vi "Asensor_parccial.vi"() -> ()   [LabVIEW 2019]
panel:
  in  "Abierto/Cerrado":bool=TRUE
  in  "Sensor":bool
  out "Indicador_Piso":u16(ring)
  in  "Botonera 3":bool
  in  "Botonera 4":bool
  in  "Botonera 1":bool
  in  "Botonera 2":bool
  in  "Peticion_Abrir":bool
  in  "Peticion_Cerrar":bool
  in  "Subir/Bajar":bool
  in  "Automatico/Manual":bool
  in  "Start/Stop":bool
  in  "Piso inicial":i32=1 min=1 max=4
  out "Numeric 2":u8
  out "Numeric":i32
  out "Subiendo":bool
  out "Bajando":bool
  out "Sensor 4":bool
  out "Sensor 3":bool
  out "Sensor 2":bool
  out "Sensor 1":bool
  in  "Piso 3_Bajar":bool
  in  "Piso 3_Subir":bool
  in  "Piso 2_Bajar":bool
  in  "Piso 2_Subir":bool
  in  "Piso 1_Subir":bool
  in  "Piso 4_Bajar":bool
  out "Puerta":i32(ring)
  out "Posicion_asensor":i32(slide) scale=100.0..400.0
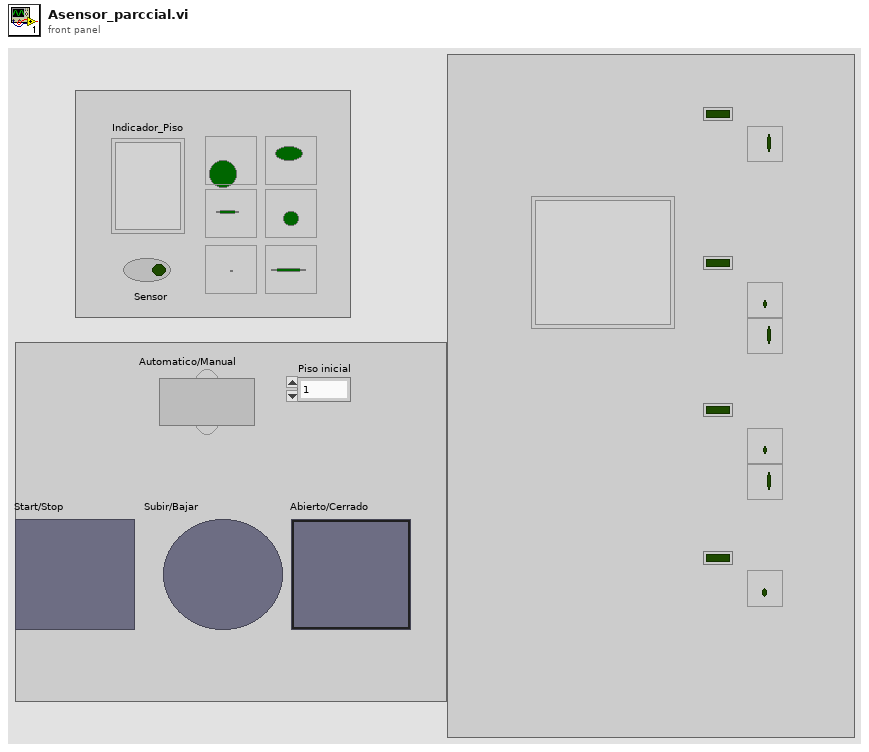
[diagram p1: front panel]
types:
  T1 = enum16{"espera", "abrir", "cerrar", "subir", "bajar"}
  T2 = enum8{"Enabled", "Disabled", "Disabled and Grayed Out"}
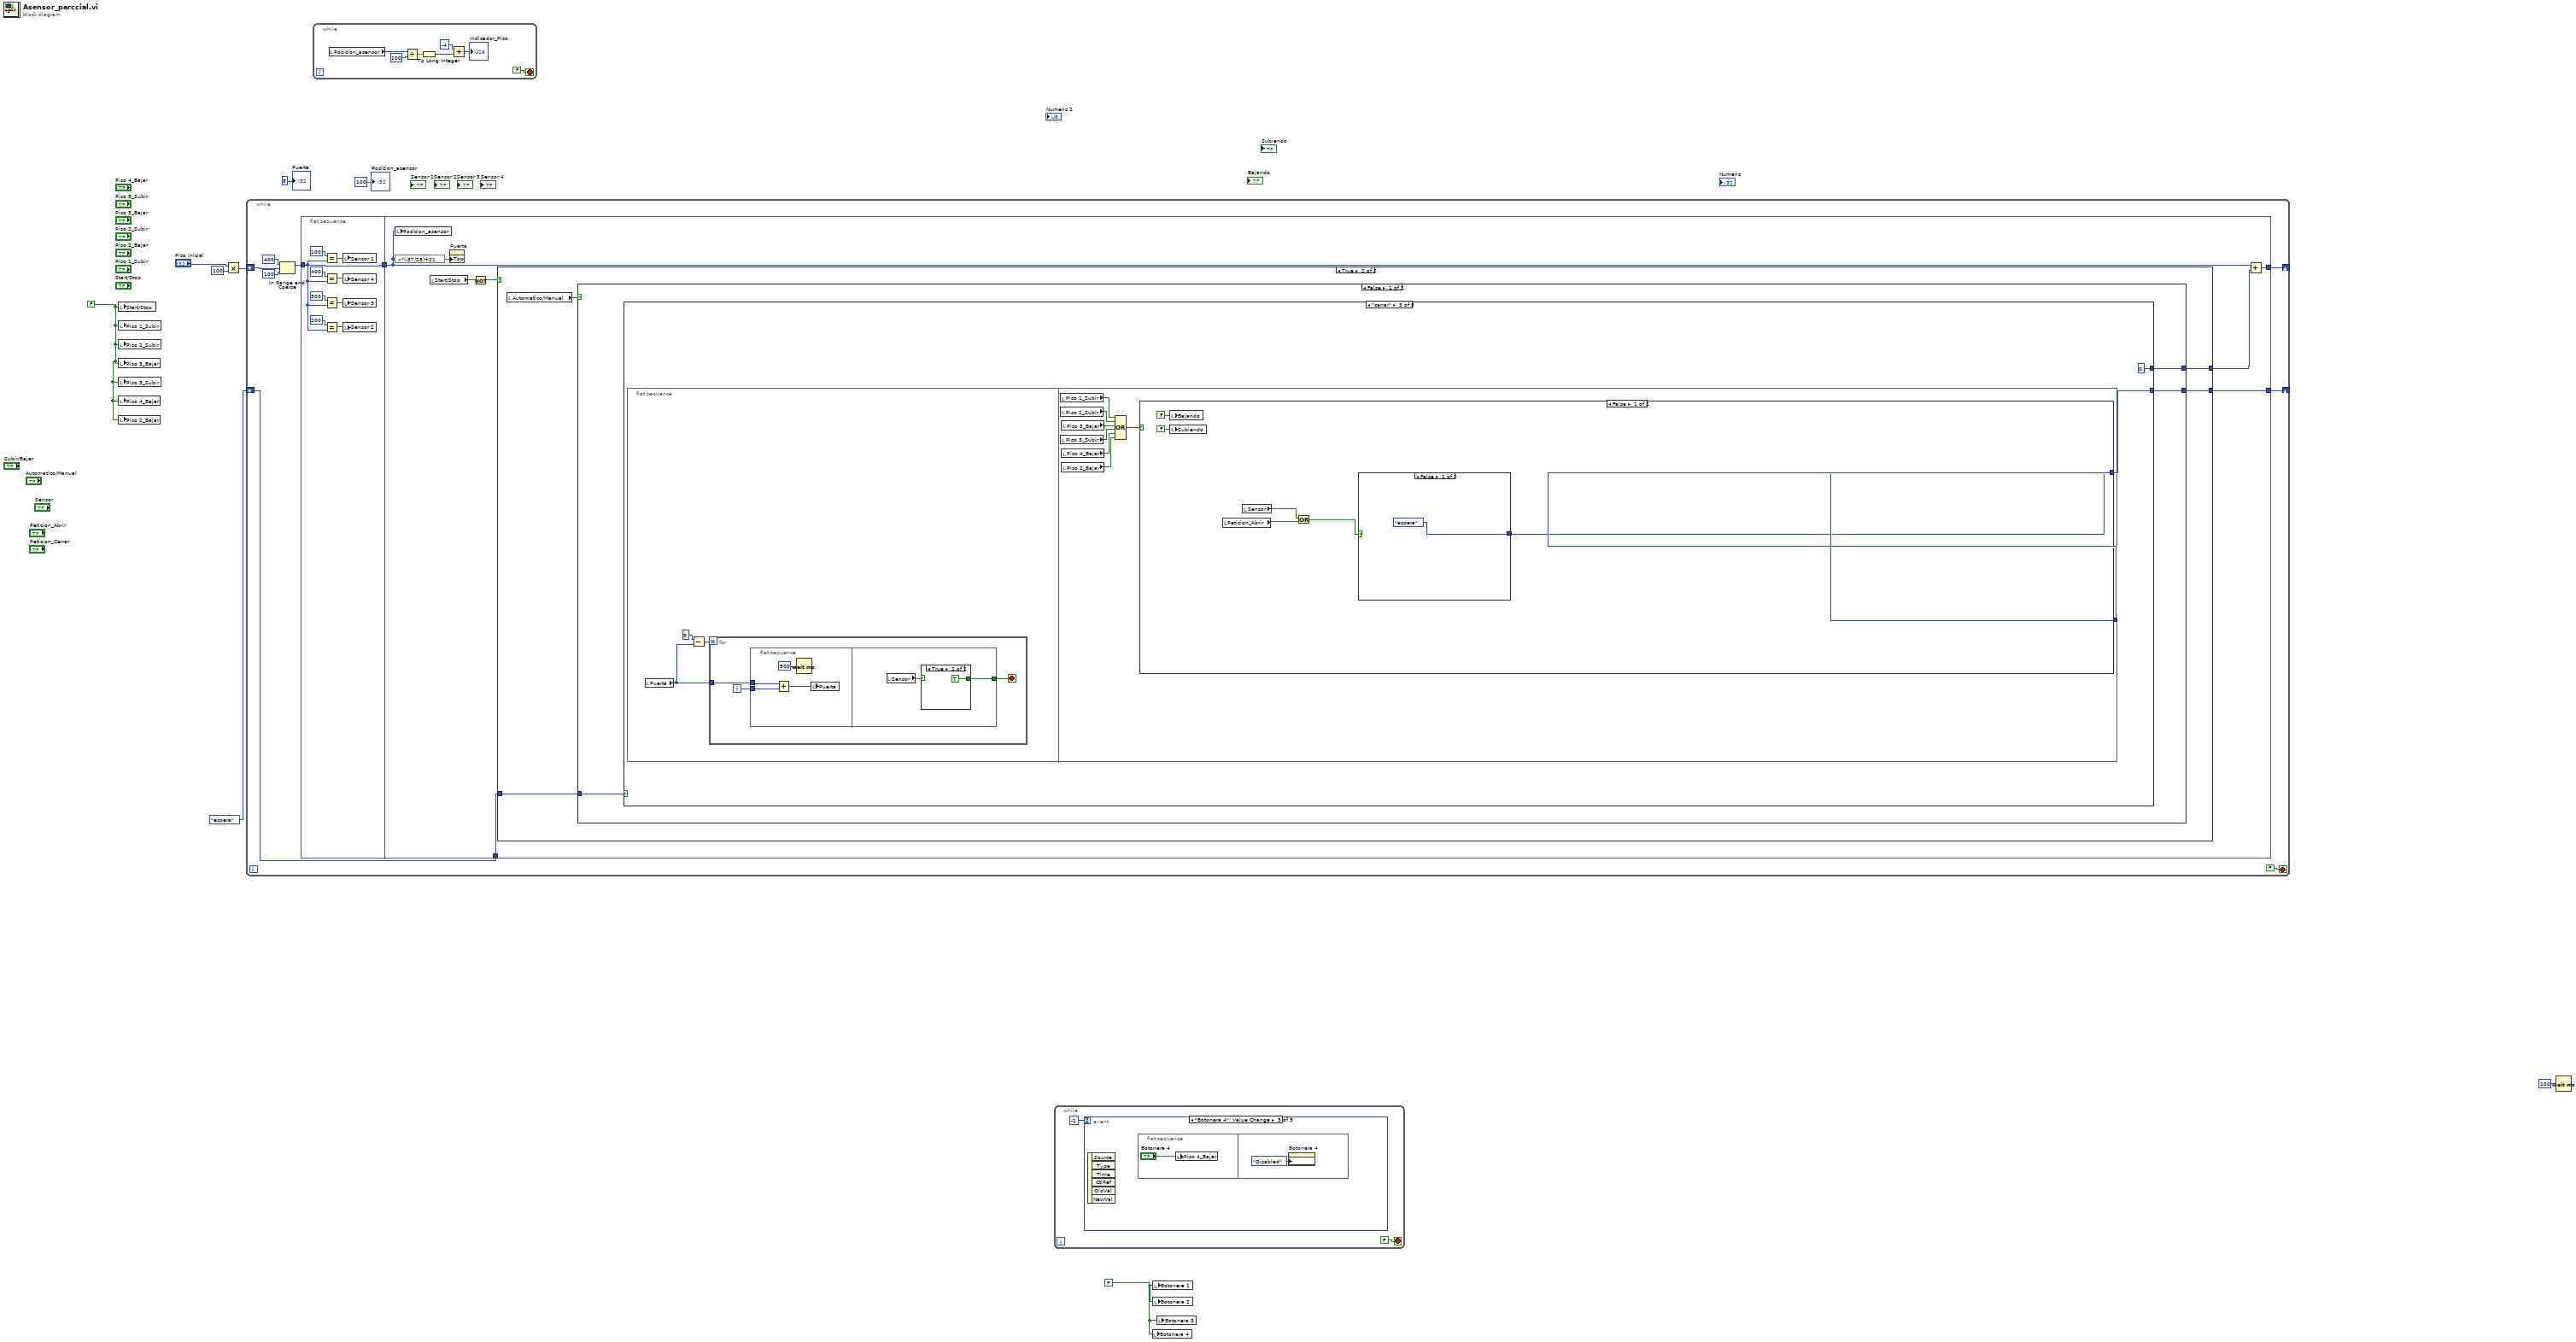
[diagram p0: block diagram]
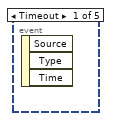
[diagram p2: hidden frame]
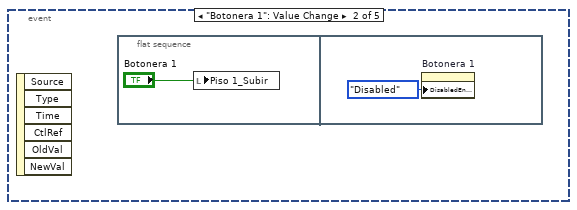
[diagram p3: hidden frame]
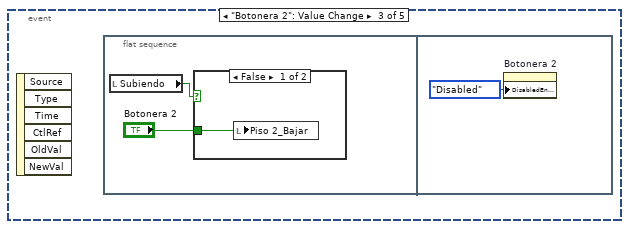
[diagram p4: hidden frame]
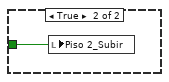
[diagram p5: hidden frame]
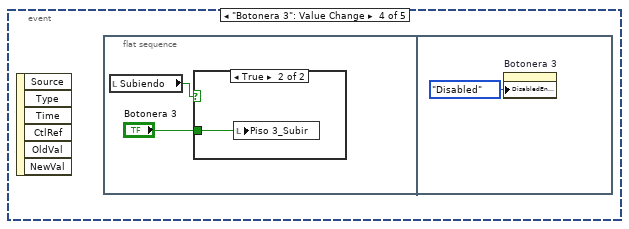
[diagram p6: hidden frame]
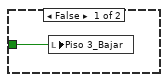
[diagram p7: hidden frame]
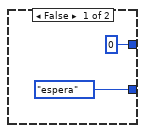
[diagram p8: hidden frame]
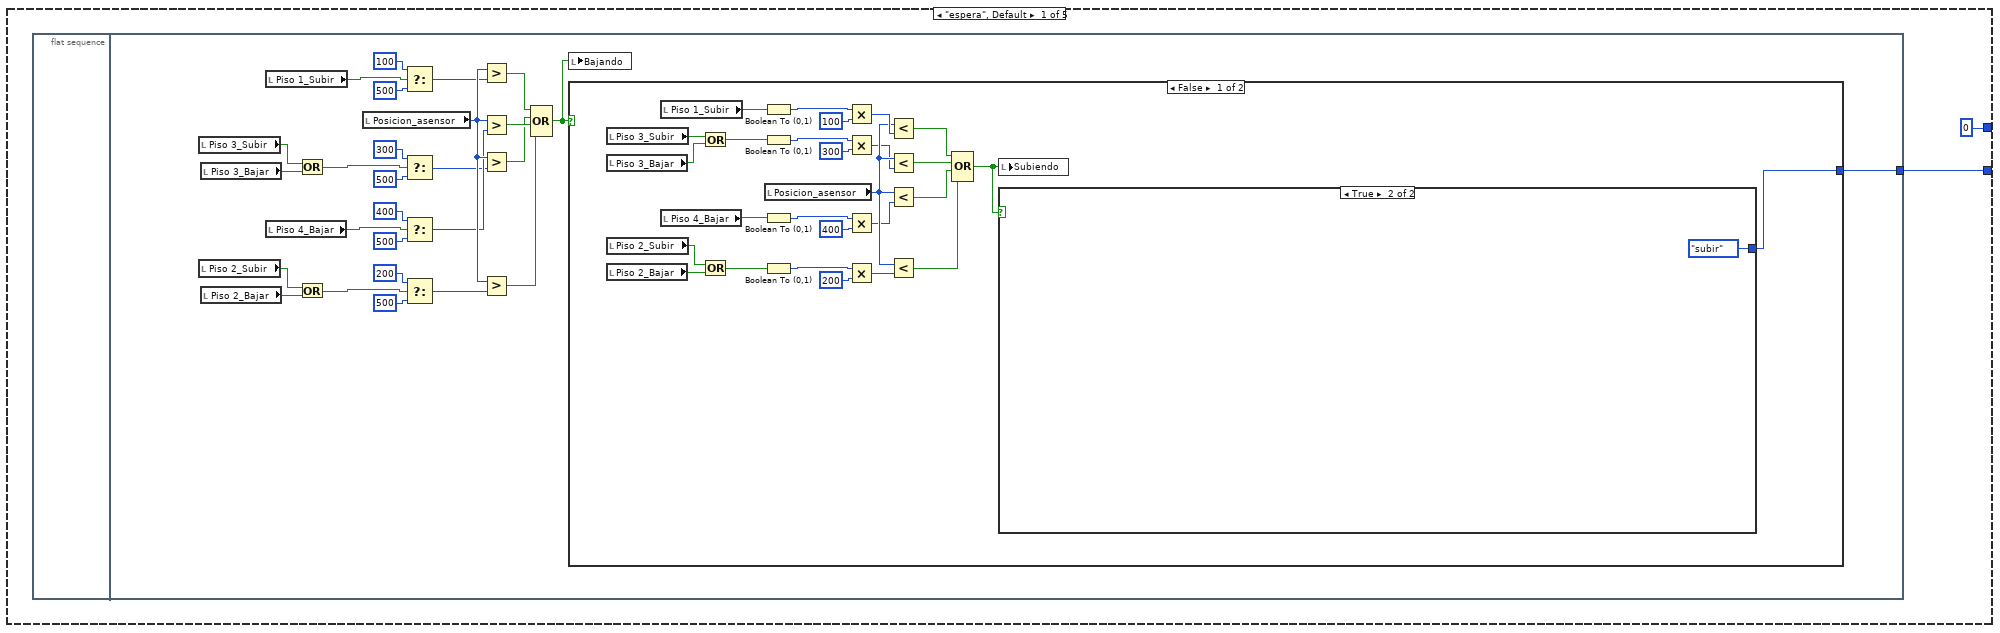
[diagram p9: hidden frame]
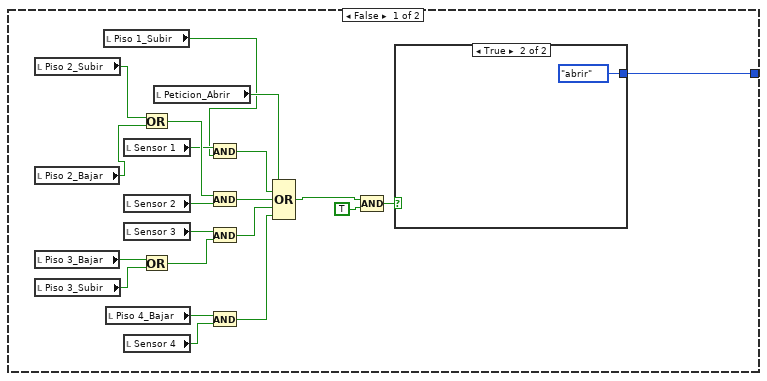
[diagram p10: hidden frame]
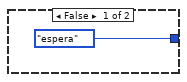
[diagram p11: hidden frame]
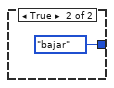
[diagram p12: hidden frame]
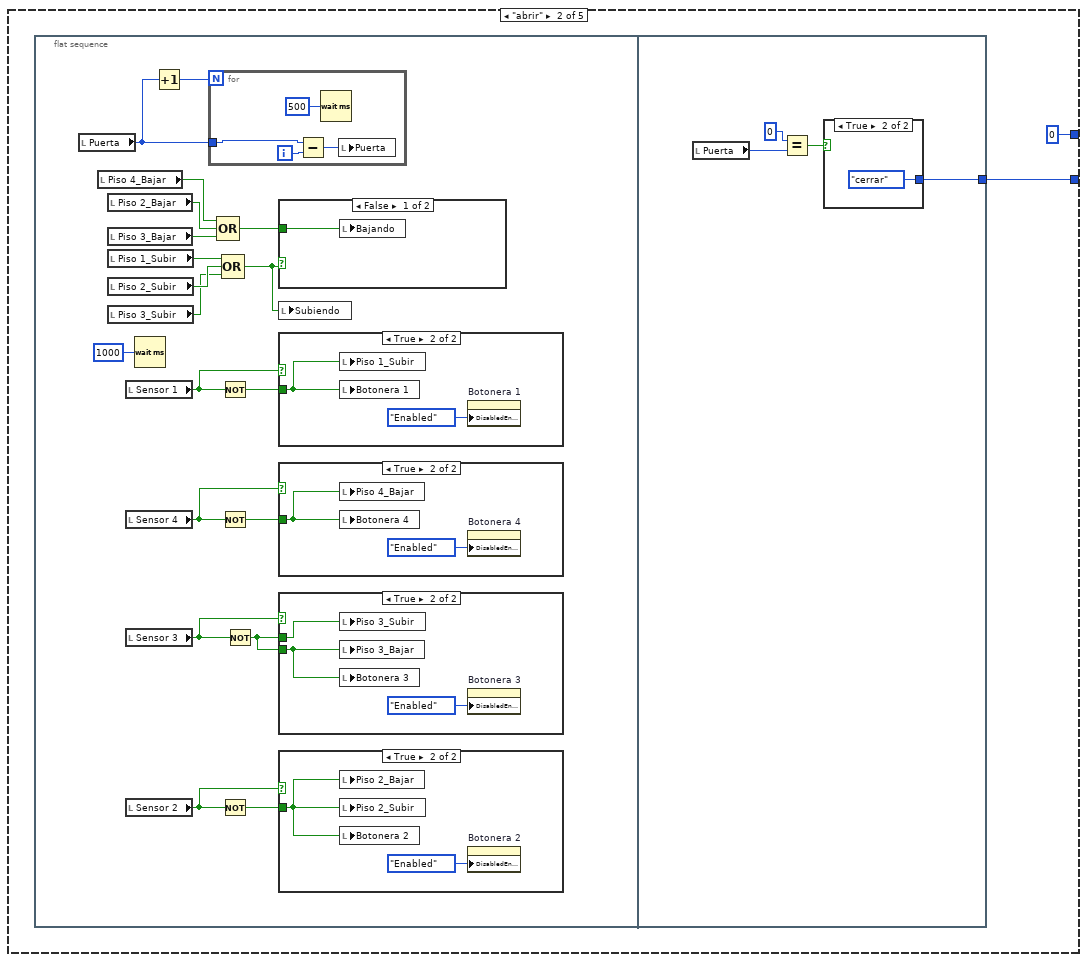
[diagram p13: hidden frame]
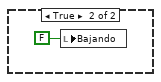
[diagram p18: hidden frame]
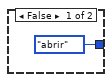
[diagram p19: hidden frame]
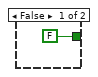
[diagram p20: hidden frame]
diagram:
  w3 = FALSE ("Botonera 1")
  w4 = FALSE ("Start/Stop")
  n1 = local write "Start/Stop"(w4) -> ()
  n2 = local write "Piso 1_Subir"(w4) -> ()
  n3 = local write "Piso 2_Subir"(w4) -> ()
  n4 = local write "Piso 3_Bajar"(w4) -> ()
  n5 = local write "Piso 3_Subir"(w4) -> ()
  n6 = local write "Piso 4_Bajar"(w4) -> ()
  n7 = local write "Piso 2_Bajar"(w4) -> ()
  n8 = Multiply(x="Piso inicial", y=100) -> (x*y=w7:i32)
  n9 = while {
    shift-right: [w12] -> _
    shift-left: w7 -> [w13]
    shift-right: [w11] -> _
    shift-left: T1."espera" -> [w10]
    stop <- FALSE stop-if-true
    n10 = In Range and Coerce(upper limit=400 ("x"), x=w13, lower limit=100 ("x")) -> (coerced(x)=w14:i32)  [unwired: 1 out]
    n11 = flat-sequence {
      tunnel: w14 -> [w23]
      tunnel: [w23] -> w17
      tunnel: w17 -> [w33]
      tunnel: [w34] -> w12
      tunnel: [w32] -> w11
      tunnel: w10 -> [w31]
      frame #0 {
        n12 = Equal?(x=100, y=w23) -> (x = y?=w19:bool)
        n13 = Equal?(x=400, y=w23) -> (x = y?=w22:bool)
        n14 = Equal?(x=300, y=w23) -> (x = y?=w21:bool)
        n15 = Equal?(x=200, y=w23) -> (x = y?=w20:bool)
        n16 = local write "Sensor 1"(w19) -> ()
        n17 = local write "Sensor 4"(w22) -> ()
        n18 = local write "Sensor 3"(w21) -> ()
        n19 = local write "Sensor 2"(w20) -> ()
      }
      frame #1 {
        n20 = local write "Posicion_asensor"(w33) -> ()
        n21 = expression code="x*(-37/25)+21"(w33) -> (w35:i32)
        n22 = local read "Start/Stop"() -> (w30:bool)
        n23 = property on="Puerta" class="Ring (strict)"("Top"=w35) -> ()  [unwired: 2 in, 2 out]
        n24 = Not(x=w30) -> (.not. x?=w29:bool)
        n25 = case shown="True" w29 {
          tunnel: [0 ("f") w40] -> w28
          tunnel: [T1."espera" w39] -> w32
          tunnel: w31 -> [_ w38]
          frame False {
          }
          frame True {
            n26 = local read "Automatico/Manual"() -> (w41:bool)
            n27 = case shown="False" w41 {
              tunnel: [w44 w463] -> w40
              tunnel: [w43 T1."espera"] -> w39
              tunnel: w38 -> [w42 _]
              frame False {
                n28 = case shown="\"cerrar\"" w42 {
                  tunnel: [0 0 0 w321 w390] -> w44
                  tunnel: [w45 w126 w168 w339 w391] -> w43
                  frame "espera", Default {
                    n29 = flat-sequence {
                      tunnel: [w47] -> w45
                      frame #0 {
                      }
                      frame #1 {
                        n30 = local read "Piso 3_Subir"() -> (w57:bool)
                        n31 = local read "Piso 2_Subir"() -> (w60:bool)
                        n32 = local read "Piso 3_Bajar"() -> (w58:bool)
                        n33 = local read "Piso 2_Bajar"() -> (w59:bool)
                        n34 = local read "Piso 1_Subir"() -> (w61:bool)
                        n35 = local read "Piso 4_Bajar"() -> (w63:bool)
                        n36 = Or(x=w57, y=w58) -> (x .or. y?=w64:bool)
                        n37 = Or(x=w60, y=w59) -> (x .or. y?=w62:bool)
                        n38 = local read "Posicion_asensor"() -> (w69:i32)
                        n39 = Select(t=100, s=w61, f=500) -> (s? t:f=w65:i32)
                        n40 = Select(t=300, s=w64, f=500) -> (s? t:f=w66:i32)
                        n41 = Select(t=400, s=w63, f=500) -> (s? t:f=w67:i32)
                        n42 = Select(t=200, s=w62, f=500) -> (s? t:f=w68:i32)
                        n43 = Greater?(x=w69, y=w65) -> (0:w70:bool)
                        n44 = Greater?(x=w69, y=w67) -> (0:w72:bool)
                        n45 = Greater?(x=w69, y=w66) -> (0:w71:bool)
                        n46 = Greater?(x=w69, y=w68) -> (0:w73:bool)
                        n47 = Compound Arithmetic op=OR(w70, w71, w72, w73) -> (w48:bool)
                        n48 = local write "Bajando"(w48) -> ()
                        n49 = case shown="False" w48 {
                          tunnel: [w74 T1."bajar"] -> w47
                          frame False {
                            n50 = local read "Piso 3_Subir"() -> (w97:bool)
                            n51 = local read "Piso 3_Bajar"() -> (w98:bool)
                            n52 = local read "Piso 2_Subir"() -> (w100:bool)
                            n53 = local read "Piso 2_Bajar"() -> (w99:bool)
                            n54 = local read "Piso 1_Subir"() -> (w94:bool)
                            n55 = local read "Piso 4_Bajar"() -> (w93:bool)
                            n56 = Or(x=w97, y=w98) -> (x .or. y?=w96:bool)
                            n57 = Or(x=w100, y=w99) -> (x .or. y?=w95:bool)
                            n58 = Boolean To (0,1)(Boolean=w94) -> (0, 1=w92:i16)
                            n59 = Boolean To (0,1)(Boolean=w96) -> (0, 1=w90:i16)
                            n60 = Boolean To (0,1)(Boolean=w93) -> (0, 1=w89:i16)
                            n61 = Boolean To (0,1)(Boolean=w95) -> (0, 1=w91:i16)
                            n62 = local read "Posicion_asensor"() -> (w87:i32)
                            n63 = Multiply(x=w92, y=i16 100) -> (x*y=w88:i16)
                            n64 = Multiply(x=w90, y=i16 300) -> (x*y=w86:i16)
                            n65 = Multiply(x=w89, y=i16 400) -> (x*y=w85:i16)
                            n66 = Multiply(x=w91, y=i16 200) -> (x*y=w84:i16)
                            n67 = Less?(x=w87, y=w88) -> (x < y?=w80:bool)
                            n68 = Less?(x=w87, y=w86) -> (x < y?=w81:bool)
                            n69 = Less?(x=w87, y=w85) -> (x < y?=w82:bool)
                            n70 = Less?(x=w87, y=w84) -> (x < y?=w83:bool)
                            n71 = Compound Arithmetic op=OR(w80, w81, w82, w83) -> (w75:bool)
                            n72 = local write "Subiendo"(w75) -> ()
                            n73 = case shown="True" w75 {
                              tunnel: [w102 T1."subir"] -> w74
                              frame False {
                                n74 = local read "Piso 2_Subir"() -> (w104:bool)
                                n75 = local read "Piso 2_Bajar"() -> (w105:bool)
                                n76 = local read "Piso 3_Bajar"() -> (w106:bool)
                                n77 = local read "Piso 3_Subir"() -> (w107:bool)
                                n78 = local read "Piso 1_Subir"() -> (w108:bool)
                                n79 = local read "Piso 4_Bajar"() -> (w115:bool)
                                n80 = local read "Sensor 1"() -> (w109:bool)
                                n81 = local read "Sensor 2"() -> (w111:bool)
                                n82 = local read "Sensor 3"() -> (w112:bool)
                                n83 = local read "Sensor 4"() -> (w114:bool)
                                n84 = Or(x=w104, y=w105) -> (x .or. y?=w110:bool)
                                n85 = Or(x=w106, y=w107) -> (x .or. y?=w113:bool)
                                n86 = local read "Peticion_Abrir"() -> (w120:bool)
                                n87 = And(x=w109, y=w108) -> (x .and. y?=w119:bool)
                                n88 = And(x=w110, y=w111) -> (x .and. y?=w118:bool)
                                n89 = And(x=w112, y=w113) -> (x .and. y?=w117:bool)
                                n90 = And(x=w115, y=w114) -> (x .and. y?=w116:bool)
                                n91 = Compound Arithmetic op=OR(w120, w119, w118, w117, w116) -> (w121:bool)
                                n92 = Compound Arithmetic op=AND(w121, TRUE ("value")) -> (w103:bool)
                                n93 = case shown="True" w103 {
                                tunnel: [T1."espera" T1."abrir"] -> w102
                                frame False {
                                }
                                frame True {
                                }
                                }
                              }
                              frame True {
                              }
                            }
                          }
                          frame True {
                          }
                        }
                      }
                    }
                  }
                  frame "abrir" {
                    n94 = flat-sequence {
                      tunnel: [w162] -> w126
                      frame #0 {
                        n95 = local read "Puerta"() -> (w128:i32)
                        n96 = local read "Piso 4_Bajar"() -> (w142:bool)
                        n97 = local read "Piso 2_Bajar"() -> (w141:bool)
                        n98 = local read "Piso 3_Bajar"() -> (w140:bool)
                        n99 = local read "Piso 1_Subir"() -> (w145:bool)
                        n100 = local read "Piso 2_Subir"() -> (w144:bool)
                        n101 = local read "Piso 3_Subir"() -> (w143:bool)
                        n102 = local read "Sensor 1"() -> (w137:bool)
                        n103 = local read "Sensor 4"() -> (w136:bool)
                        n104 = local read "Sensor 3"() -> (w135:bool)
                        n105 = local read "Sensor 2"() -> (w134:bool)
                        n106 = Wait (ms)(milliseconds to wait=u32 1000) -> ()  [unwired: 1 out]
                        n107 = Increment(x=w128) -> (x+1=w129:i32)
                        n108 = for {
                          N: w129 -> [_]
                          tunnel: w128 -> [w161]
                          i -> [w160]
                          n109 = Subtract(x=w161, y=w160) -> (x-y=w159:i32)
                          n110 = Wait (ms)(milliseconds to wait=u32 500) -> ()  [unwired: 1 out]
                          n111 = local write "Puerta"(w159) -> ()
                        }
                        n112 = Compound Arithmetic op=OR(w142, w141, w140) -> (w138:bool)
                        n113 = Not(x=w137) -> (.not. x?=w133:bool)
                        n114 = Not(x=w136) -> (.not. x?=w132:bool)
                        n115 = Not(x=w134) -> (.not. x?=w130:bool)
                        n116 = Compound Arithmetic op=OR(w145, w144, w143) -> (w139:bool)
                        n117 = Not(x=w135) -> (.not. x?=w131:bool)
                        n118 = case shown="False" w139 {
                          tunnel: w138 -> [w156 _]
                          frame False {
                            n119 = local write "Bajando"(w156) -> ()
                          }
                          frame True {
                            n120 = local write "Bajando"(FALSE ("Bajando")) -> ()
                          }
                        }
                        n121 = local write "Subiendo"(w139) -> ()
                        n122 = case shown="True" w137 {
                          tunnel: w133 -> [_ w154]
                          frame False {
                          }
                          frame True {
                            n123 = local write "Piso 1_Subir"(w154) -> ()
                            n124 = local write "Botonera 1"(w154) -> ()
                            n125 = property on="Botonera 1" class="Bool (strict)"("DisabledEnum"=T2."Enabled" ("Disabled")) -> ()  [unwired: 2 in, 2 out]
                          }
                        }
                        n126 = case shown="True" w136 {
                          tunnel: w132 -> [_ w152]
                          frame False {
                          }
                          frame True {
                            n127 = local write "Piso 4_Bajar"(w152) -> ()
                            n128 = local write "Botonera 4"(w152) -> ()
                            n129 = property on="Botonera 4" class="Bool (strict)"("DisabledEnum"=T2."Enabled" ("Disabled")) -> ()  [unwired: 2 in, 2 out]
                          }
                        }
                        n130 = case shown="True" w135 {
                          tunnel: w131 -> [_ w149]
                          tunnel: w131 -> [_ w151]
                          frame False {
                          }
                          frame True {
                            n131 = local write "Piso 3_Subir"(w151) -> ()
                            n132 = local write "Piso 3_Bajar"(w149) -> ()
                            n133 = local write "Botonera 3"(w149) -> ()
                            n134 = property on="Botonera 3" class="Bool (strict)"("DisabledEnum"=T2."Enabled" ("Disabled")) -> ()  [unwired: 2 in, 2 out]
                          }
                        }
                        n135 = case shown="True" w134 {
                          tunnel: w130 -> [_ w147]
                          frame False {
                          }
                          frame True {
                            n136 = local write "Piso 2_Bajar"(w147) -> ()
                            n137 = local write "Piso 2_Subir"(w147) -> ()
                            n138 = local write "Botonera 2"(w147) -> ()
                            n139 = property on="Botonera 2" class="Bool (strict)"("DisabledEnum"=T2."Enabled" ("Disabled")) -> ()  [unwired: 2 in, 2 out]
                          }
                        }
                      }
                      frame #1 {
                        n140 = local read "Puerta"() -> (w165:i32)
                        n141 = Equal?(x=0, y=w165) -> (x = y?=w163:bool)
                        n142 = case shown="True" w163 {
                          tunnel: [T1."abrir" T1."cerrar"] -> w162
                          frame False {
                          }
                          frame True {
                          }
                        }
                      }
                    }
                  }
                  frame "cerrar" {
                    n143 = flat-sequence {
                      tunnel: [w184] -> w168
                      frame #0 {
                        n144 = local read "Puerta"() -> (w170:i32)
                        n145 = Subtract(x=9, y=w170) -> (x-y=w171:i32)
                        n146 = for {
                          N: w171 -> [_]
                          tunnel: w170 -> [w175]
                          i -> [w174]
                          stop <- w173 stop-if-true
                          n147 = flat-sequence {
                            tunnel: w175 -> [w179]
                            tunnel: w174 -> [w178]
                            tunnel: [w180] -> w173
                            frame #0 {
                              n148 = Add(x=w179, y=w178) -> (x+y=w176:i32)
                              n149 = Wait (ms)(milliseconds to wait=u32 500) -> ()  [unwired: 1 out]
                              n150 = local write "Puerta"(w176) -> ()
                            }
                            frame #1 {
                              n151 = local read "Sensor"() -> (w181:bool)
                              n152 = case shown="True" w181 {
                                tunnel: [FALSE TRUE] -> w180
                                frame False {
                                }
                                frame True {
                                }
                              }
                            }
                          }
                        }
                      }
                      frame #1 {
                        n153 = local read "Piso 1_Subir"() -> (w185:bool)
                        n154 = local read "Piso 2_Subir"() -> (w186:bool)
                        n155 = local read "Piso 3_Subir"() -> (w188:bool)
                        n156 = local read "Piso 3_Bajar"() -> (w187:bool)
                        n157 = local read "Piso 4_Bajar"() -> (w189:bool)
                        n158 = local read "Piso 2_Bajar"() -> (w190:bool)
                        n159 = Compound Arithmetic op=OR(w185, w186, w187, w188, w189, w190) -> (w191:bool)
                        n160 = case shown="False" w191 {
                          tunnel: [w192 w200] -> w184
                          frame False {
                            n161 = local write "Bajando"(FALSE ("Bajando")) -> ()
                            n162 = local write "Subiendo"(FALSE ("Subiendo")) -> ()
                            n163 = local read "Peticion_Abrir"() -> (w195:bool)
                            n164 = local read "Sensor"() -> (w194:bool)
                            n165 = Or(x=w194, y=w195) -> (x .or. y?=w193:bool)
                            n166 = case shown="False" w193 {
                              tunnel: [T1."espera" T1."abrir"] -> w192
                              frame False {
                              }
                              frame True {
                              }
                            }
                          }
                          frame True {
                            n167 = local read "Piso 2_Subir"() -> (w218:bool)
                            n168 = local read "Piso 2_Bajar"() -> (w217:bool)
                            n169 = local read "Piso 3_Bajar"() -> (w216:bool)
                            n170 = local read "Piso 3_Subir"() -> (w215:bool)
                            n171 = local read "Piso 1_Subir"() -> (w214:bool)
                            n172 = local read "Piso 4_Bajar"() -> (w207:bool)
                            n173 = local read "Sensor 1"() -> (w213:bool)
                            n174 = local read "Sensor 2"() -> (w211:bool)
                            n175 = local read "Sensor 3"() -> (w210:bool)
                            n176 = local read "Sensor 4"() -> (w208:bool)
                            n177 = Or(x=w218, y=w217) -> (x .or. y?=w212:bool)
                            n178 = Or(x=w216, y=w215) -> (x .or. y?=w209:bool)
                            n179 = local read "Peticion_Abrir"() -> (w202:bool)
                            n180 = local read "Sensor"() -> (w219:bool)
                            n181 = And(x=w213, y=w214) -> (x .and. y?=w203:bool)
                            n182 = And(x=w212, y=w211) -> (x .and. y?=w204:bool)
                            n183 = And(x=w210, y=w209) -> (x .and. y?=w205:bool)
                            n184 = And(x=w207, y=w208) -> (x .and. y?=w206:bool)
                            n185 = Compound Arithmetic op=OR(w219, w202, w203, w204, w205, w206) -> (w201:bool)
                            n186 = case shown="True" w201 {
                              tunnel: [w220 T1."abrir"] -> w200
                              frame False {
                                n187 = local read "Subiendo"() -> (w221:bool)
                                n188 = case shown="True" w221 {
                                tunnel: [w222 w271] -> w220
                                frame False {
                                n189 = local read "Piso 1_Subir"() -> (w244:bool)
                                n190 = local read "Piso 3_Bajar"() -> (w233:bool)
                                n191 = local read "Piso 4_Bajar"() -> (w243:bool)
                                n192 = local read "Piso 2_Bajar"() -> (w232:bool)
                                n193 = local read "Posicion_asensor"() -> (w238:i32)
                                n194 = Select(t=100, s=w244, f=500) -> (s? t:f=w242:i32)
                                n195 = Select(t=300, s=w233, f=500) -> (s? t:f=w241:i32)
                                n196 = Select(t=400, s=w243, f=500) -> (s? t:f=w240:i32)
                                n197 = Select(t=200, s=w232, f=500) -> (s? t:f=w239:i32)
                                n198 = Greater?(x=w238, y=w242) -> (0:w237:bool)
                                n199 = Greater?(x=w238, y=w241) -> (0:w236:bool)
                                n200 = Greater?(x=w238, y=w240) -> (0:w235:bool)
                                n201 = Greater?(x=w238, y=w239) -> (0:w234:bool)
                                n202 = Compound Arithmetic op=OR(w237, w236, w235, w234) -> (w223:bool)
                                n203 = case shown="False" w223 {
                                tunnel: [w245 T1."bajar"] -> w222
                                frame False {
                                n204 = local read "Piso 1_Subir"() -> (w251:bool)
                                n205 = local read "Piso 3_Subir"() -> (w266:bool)
                                n206 = local read "Piso 2_Subir"() -> (w267:bool)
                                n207 = local read "Piso 4_Bajar"() -> (w252:bool)
                                n208 = local read "Posicion_asensor"() -> (w258:i32)
                                n209 = Boolean To (0,1)(Boolean=w251) -> (0, 1=w253:i16)
                                n210 = Boolean To (0,1)(Boolean=w266) -> (0, 1=w255:i16)
                                n211 = Boolean To (0,1)(Boolean=w252) -> (0, 1=w256:i16)
                                n212 = Boolean To (0,1)(Boolean=w267) -> (0, 1=w254:i16)
                                n213 = Multiply(x=w253, y=i16 100) -> (x*y=w257:i16)
                                n214 = Multiply(x=w255, y=i16 300) -> (x*y=w259:i16)
                                n215 = Multiply(x=w256, y=i16 400) -> (x*y=w260:i16)
                                n216 = Multiply(x=w254, y=i16 200) -> (x*y=w261:i16)
                                n217 = Less?(x=w258, y=w257) -> (x < y?=w265:bool)
                                n218 = Less?(x=w258, y=w259) -> (x < y?=w264:bool)
                                n219 = Less?(x=w258, y=w260) -> (x < y?=w263:bool)
                                n220 = Less?(x=w258, y=w261) -> (x < y?=w262:bool)
                                n221 = Compound Arithmetic op=OR(w265, w264, w263, w262) -> (w246:bool)
                                n222 = case shown="False" w246 {
                                tunnel: [T1."espera" T1."subir"] -> w245
                                frame False {
                                }
                                frame True {
                                }
                                }
                                }
                                frame True {
                                }
                                }
                                }
                                frame True {
                                n223 = local read "Piso 1_Subir"() -> (w277:bool)
                                n224 = local read "Piso 3_Subir"() -> (w292:bool)
                                n225 = local read "Piso 4_Bajar"() -> (w278:bool)
                                n226 = local read "Piso 2_Subir"() -> (w293:bool)
                                n227 = local read "Posicion_asensor"() -> (w284:i32)
                                n228 = Boolean To (0,1)(Boolean=w277) -> (0, 1=w279:i16)
                                n229 = Boolean To (0,1)(Boolean=w292) -> (0, 1=w281:i16)
                                n230 = Boolean To (0,1)(Boolean=w278) -> (0, 1=w282:i16)
                                n231 = Boolean To (0,1)(Boolean=w293) -> (0, 1=w280:i16)
                                n232 = Multiply(x=w279, y=i16 100) -> (x*y=w283:i16)
                                n233 = Multiply(x=w281, y=i16 300) -> (x*y=w285:i16)
                                n234 = Multiply(x=w282, y=i16 400) -> (x*y=w286:i16)
                                n235 = Multiply(x=w280, y=i16 200) -> (x*y=w287:i16)
                                n236 = Less?(x=w284, y=w283) -> (x < y?=w291:bool)
                                n237 = Less?(x=w284, y=w285) -> (x < y?=w290:bool)
                                n238 = Less?(x=w284, y=w286) -> (x < y?=w289:bool)
                                n239 = Less?(x=w284, y=w287) -> (x < y?=w288:bool)
                                n240 = Compound Arithmetic op=OR(w291, w290, w289, w288) -> (w272:bool)
                                n241 = case shown="False" w272 {
                                tunnel: [w294 T1."subir"] -> w271
                                frame False {
                                n242 = local read "Piso 1_Subir"() -> (w316:bool)
                                n243 = local read "Piso 3_Bajar"() -> (w297:bool)
                                n244 = local read "Piso 4_Bajar"() -> (w315:bool)
                                n245 = local read "Piso 2_Bajar"() -> (w296:bool)
                                n246 = local read "Posicion_asensor"() -> (w310:i32)
                                n247 = Select(t=100, s=w316, f=500) -> (s? t:f=w314:i32)
                                n248 = Select(t=300, s=w297, f=500) -> (s? t:f=w313:i32)
                                n249 = Select(t=400, s=w315, f=500) -> (s? t:f=w312:i32)
                                n250 = Select(t=200, s=w296, f=500) -> (s? t:f=w311:i32)
                                n251 = Greater?(x=w310, y=w314) -> (0:w309:bool)
                                n252 = Greater?(x=w310, y=w313) -> (0:w308:bool)
                                n253 = Greater?(x=w310, y=w312) -> (0:w307:bool)
                                n254 = Greater?(x=w310, y=w311) -> (0:w306:bool)
                                n255 = Compound Arithmetic op=OR(w309, w308, w307, w306) -> (w298:bool)
                                n256 = case shown="True" w298 {
                                tunnel: [T1."espera" T1."bajar"] -> w294
                                frame False {
                                }
                                frame True {
                                }
                                }
                                }
                                frame True {
                                }
                                }
                                }
                                }
                              }
                              frame True {
                              }
                            }
                          }
                        }
                      }
                    }
                  }
                  frame "subir" {
                    n257 = local write "Subiendo"(TRUE ("Subiendo")) -> ()
                    n258 = local write "Bajando"(FALSE ("Bajando")) -> ()
                    n259 = Wait (ms)(milliseconds to wait=u32 100) -> ()  [unwired: 1 out]
                    n260 = local read "Piso 2_Subir"() -> (w338:bool)
                    n261 = local read "Piso 2_Bajar"() -> (w337:bool)
                    n262 = local read "Piso 3_Bajar"() -> (w336:bool)
                    n263 = local read "Piso 3_Subir"() -> (w335:bool)
                    n264 = local read "Piso 1_Subir"() -> (w324:bool)
                    n265 = local read "Piso 4_Bajar"() -> (w333:bool)
                    n266 = local read "Sensor 1"() -> (w323:bool)
                    n267 = local read "Sensor 2"() -> (w328:bool)
                    n268 = local read "Sensor 3"() -> (w330:bool)
                    n269 = local read "Sensor 4"() -> (w332:bool)
                    n270 = Or(x=w338, y=w337) -> (x .or. y?=w329:bool)
                    n271 = Or(x=w336, y=w335) -> (x .or. y?=w331:bool)
                    n272 = And(x=w324, y=w323) -> (x .and. y?=w322:bool)
                    n273 = And(x=w329, y=w328) -> (x .and. y?=w327:bool)
                    n274 = And(x=w330, y=w331) -> (x .and. y?=w325:bool)
                    n275 = And(x=w333, y=w332) -> (x .and. y?=w326:bool)
                    n276 = Compound Arithmetic op=OR(w322, w327, w325, w326) -> (w334:bool)
                    n277 = case shown="True" w334 {
                      tunnel: [T1."subir" w351] -> w339
                      tunnel: [1 w349] -> w321
                      frame False {
                      }
                      frame True {
                        n278 = local read "Piso 1_Subir"() -> (w348:bool)
                        n279 = local read "Piso 2_Subir"() -> (w347:bool)
                        n280 = local read "Piso 3_Subir"() -> (w346:bool)
                        n281 = local read "Piso 4_Bajar"() -> (w345:bool)
                        n282 = Compound Arithmetic op=OR(w348, w347, w346, w345) -> (w350:bool)
                        n283 = case shown="True" w350 {
                          tunnel: [w353 w372] -> w351
                          tunnel: [w352 w371] -> w349
                          frame False {
                            n284 = local read "Piso 1_Subir"() -> (w357:bool)
                            n285 = local read "Piso 2_Bajar"() -> (w365:bool)
                            n286 = local read "Piso 3_Bajar"() -> (w366:bool)
                            n287 = local read "Piso 4_Bajar"() -> (w364:bool)
                            n288 = local read "Sensor 1"() -> (w356:bool)
                            n289 = local read "Sensor 2"() -> (w361:bool)
                            n290 = local read "Sensor 3"() -> (w362:bool)
                            n291 = local read "Sensor 4"() -> (w363:bool)
                            n292 = And(x=w357, y=w356) -> (x .and. y?=w355:bool)
                            n293 = And(x=w365, y=w361) -> (x .and. y?=w360:bool)
                            n294 = And(x=w362, y=w366) -> (x .and. y?=w358:bool)
                            n295 = And(x=w364, y=w363) -> (x .and. y?=w359:bool)
                            n296 = Compound Arithmetic op=OR(w355, w360, w358, w359) -> (w354:bool)
                            n297 = case shown="False" w354 {
                              tunnel: [T1."subir" T1."abrir"] -> w353
                              tunnel: [1 0] -> w352
                              frame False {
                              }
                              frame True {
                              }
                            }
                          }
                          frame True {
                            n298 = local read "Piso 1_Subir"() -> (w383:bool)
                            n299 = local read "Piso 2_Subir"() -> (w374:bool)
                            n300 = local read "Piso 3_Subir"() -> (w375:bool)
                            n301 = local read "Piso 4_Bajar"() -> (w376:bool)
                            n302 = local read "Sensor 1"() -> (w384:bool)
                            n303 = local read "Sensor 2"() -> (w379:bool)
                            n304 = local read "Sensor 3"() -> (w378:bool)
                            n305 = local read "Sensor 4"() -> (w377:bool)
                            n306 = And(x=w383, y=w384) -> (x .and. y?=w385:bool)
                            n307 = And(x=w374, y=w379) -> (x .and. y?=w380:bool)
                            n308 = And(x=w378, y=w375) -> (x .and. y?=w382:bool)
                            n309 = And(x=w376, y=w377) -> (x .and. y?=w381:bool)
                            n310 = Compound Arithmetic op=OR(w385, w380, w382, w381) -> (w373:bool)
                            n311 = case shown="False" w373 {
                              tunnel: [T1."subir" T1."abrir"] -> w372
                              tunnel: [1 0] -> w371
                              frame False {
                              }
                              frame True {
                              }
                            }
                          }
                        }
                      }
                    }
                  }
                  frame "bajar" {
                    n312 = local write "Subiendo"(FALSE ("Subiendo")) -> ()
                    n313 = local write "Bajando"(TRUE ("Bajando")) -> ()
                    n314 = Wait (ms)(milliseconds to wait=u32 100) -> ()  [unwired: 1 out]
                    n315 = local read "Piso 2_Subir"() -> (w410:bool)
                    n316 = local read "Piso 2_Bajar"() -> (w409:bool)
                    n317 = local read "Piso 3_Bajar"() -> (w408:bool)
                    n318 = local read "Piso 3_Subir"() -> (w407:bool)
                    n319 = local read "Piso 1_Subir"() -> (w406:bool)
                    n320 = local read "Piso 4_Bajar"() -> (w399:bool)
                    n321 = local read "Sensor 1"() -> (w405:bool)
                    n322 = local read "Sensor 2"() -> (w403:bool)
                    n323 = local read "Sensor 3"() -> (w402:bool)
                    n324 = local read "Sensor 4"() -> (w400:bool)
                    n325 = Or(x=w410, y=w409) -> (x .or. y?=w404:bool)
                    n326 = Or(x=w408, y=w407) -> (x .or. y?=w401:bool)
                    n327 = And(x=w405, y=w406) -> (x .and. y?=w398:bool)
                    n328 = And(x=w404, y=w403) -> (x .and. y?=w397:bool)
                    n329 = And(x=w402, y=w401) -> (x .and. y?=w396:bool)
                    n330 = And(x=w399, y=w400) -> (x .and. y?=w395:bool)
                    n331 = Compound Arithmetic op=OR(w398, w397, w396, w395) -> (w394:bool)
                    n332 = case shown="True" w394 {
                      tunnel: [w416 T1."bajar"] -> w391
                      tunnel: [w417 -1] -> w390
                      frame True {
                        n333 = local read "Piso 1_Subir"() -> (w415:bool)
                        n334 = local read "Piso 2_Bajar"() -> (w414:bool)
                        n335 = local read "Piso 3_Bajar"() -> (w413:bool)
                        n336 = local read "Piso 4_Bajar"() -> (w412:bool)
                        n337 = Compound Arithmetic op=OR(w415, w414, w413, w412) -> (w418:bool)
                        n338 = case shown="True" w418 {
                          tunnel: [w419 w438] -> w417
                          tunnel: [w420 w439] -> w416
                          frame False {
                            n339 = local read "Piso 1_Subir"() -> (w431:bool)
                            n340 = local read "Piso 2_Subir"() -> (w433:bool)
                            n341 = local read "Piso 3_Subir"() -> (w432:bool)
                            n342 = local read "Piso 4_Bajar"() -> (w426:bool)
                            n343 = local read "Sensor 1"() -> (w430:bool)
                            n344 = local read "Sensor 2"() -> (w429:bool)
                            n345 = local read "Sensor 3"() -> (w428:bool)
                            n346 = local read "Sensor 4"() -> (w427:bool)
                            n347 = And(x=w430, y=w431) -> (x .and. y?=w425:bool)
                            n348 = And(x=w433, y=w429) -> (x .and. y?=w424:bool)
                            n349 = And(x=w428, y=w432) -> (x .and. y?=w423:bool)
                            n350 = And(x=w426, y=w427) -> (x .and. y?=w422:bool)
                            n351 = Compound Arithmetic op=OR(w425, w424, w423, w422) -> (w421:bool)
                            n352 = case shown="True" w421 {
                              tunnel: [T1."bajar" T1."subir"] -> w420
                              tunnel: [-1 0] -> w419
                              frame False {
                              }
                              frame True {
                              }
                            }
                          }
                          frame True {
                            n353 = local read "Piso 1_Subir"() -> (w443:bool)
                            n354 = local read "Piso 2_Bajar"() -> (w452:bool)
                            n355 = local read "Piso 3_Bajar"() -> (w451:bool)
                            n356 = local read "Piso 4_Bajar"() -> (w450:bool)
                            n357 = local read "Sensor 1"() -> (w442:bool)
                            n358 = local read "Sensor 2"() -> (w447:bool)
                            n359 = local read "Sensor 3"() -> (w448:bool)
                            n360 = local read "Sensor 4"() -> (w449:bool)
                            n361 = And(x=w443, y=w442) -> (x .and. y?=w441:bool)
                            n362 = And(x=w452, y=w447) -> (x .and. y?=w446:bool)
                            n363 = And(x=w448, y=w451) -> (x .and. y?=w444:bool)
                            n364 = And(x=w450, y=w449) -> (x .and. y?=w445:bool)
                            n365 = Compound Arithmetic op=OR(w441, w446, w444, w445) -> (w440:bool)
                            n366 = case shown="False" w440 {
                              tunnel: [T1."bajar" T1."abrir"] -> w439
                              tunnel: [-1 0] -> w438
                              frame False {
                              }
                              frame True {
                              }
                            }
                          }
                        }
                      }
                      frame False {
                      }
                    }
                  }
                }
              }
              frame True {
                n367 = Not(x="Abierto/Cerrado") -> (.not. x?=w459:bool)
                n368 = case shown="False" w459 {
                  frame False {
                    n369 = local read "Puerta"() -> (w469:i32)
                    n370 = Subtract(x=9, y=w469) -> (x-y=w468:i32)
                    n371 = for {
                      N: w468 -> [_]
                      tunnel: w469 -> [w472]
                      i -> [w471]
                      stop <- w470 stop-if-true
                      n372 = flat-sequence {
                        tunnel: w472 -> [w476]
                        tunnel: w471 -> [w475]
                        tunnel: [w477] -> w470
                        frame #0 {
                          n373 = Add(x=w476, y=w475) -> (x+y=w473:i32)
                          n374 = Wait (ms)(milliseconds to wait=u32 200) -> ()  [unwired: 1 out]
                          n375 = local write "Puerta"(w473) -> ()
                        }
                        frame #1 {
                          n376 = local read "Sensor"() -> (w478:bool)
                          n377 = case shown="False" w478 {
                            tunnel: [FALSE TRUE] -> w477
                            frame False {
                            }
                            frame True {
                            }
                          }
                        }
                      }
                    }
                  }
                  frame True {
                    n378 = local read "Puerta"() -> (w481:i32)
                    n379 = Increment(x=w481) -> (x+1=w482:i32)
                    n380 = for {
                      N: w482 -> [_]
                      tunnel: w481 -> [w486]
                      i -> [w485]
                      n381 = Subtract(x=w486, y=w485) -> (x-y=w484:i32)
                      n382 = Wait (ms)(milliseconds to wait=u32 500) -> ()  [unwired: 1 out]
                      n383 = local write "Puerta"(w484) -> ()
                    }
                  }
                }
                n384 = Wait (ms)(milliseconds to wait=u32 100) -> ()  [unwired: 1 out]
                n385 = local read "Subir/Bajar"() -> (w466:bool)
                n386 = Select(t=1, s=w466, f=-1) -> (s? t:f=w463:i32)
              }
            }
          }
        }
        n387 = Add(x=w33, y=w28) -> (x+y=w34:i32)
      }
    }
  }
  n388 = while {
    stop <- FALSE stop-if-true
    n389 = local read "Posicion_asensor"() -> (w492:i32)
    n390 = Divide(x=w492, y=100) -> (x/y=w490:dbl)
    n391 = To Long Integer(number=w490) -> (32bit integer=w489:i32)
    n392 = Add(x=-4, y=w489) -> (x+y=→"Indicador_Piso":i32)
  }
  n393 = while {
    stop <- FALSE stop-if-true
    n394 = event shown="[4] \"Botonera 4\": Value Change" {
      selector: _ -> [_ _ _ _ _]
      dyn-events: _ -> [_ _ _ _ _]
      timeout: -1 -> [_ _ _ _ _]
      event Timeout {
        n395 = event-data() -> ()  [unwired: 1 in, 3 out]
      }
      event "Botonera 1": Value Change {
        n396 = event-data() -> ()  [unwired: 1 in, 6 out]
        n397 = flat-sequence {
          frame #0 {
            n398 = local write "Piso 1_Subir"("Botonera 1") -> ()
          }
          frame #1 {
            n399 = property on="Botonera 1" class="Bool (strict)"("DisabledEnum"=T2."Disabled" ("Disabled")) -> ()  [unwired: 2 in, 2 out]
          }
        }
      }
      event "Botonera 2": Value Change {
        n400 = event-data() -> ()  [unwired: 1 in, 6 out]
        n401 = flat-sequence {
          frame #0 {
            n402 = local read "Subiendo"() -> (w499:bool)
            n403 = case shown="False" w499 {
              tunnel: "Botonera 2" -> [w500 w501]
              frame False {
                n404 = local write "Piso 2_Bajar"(w500) -> ()
              }
              frame True {
                n405 = local write "Piso 2_Subir"(w501) -> ()
              }
            }
          }
          frame #1 {
            n406 = property on="Botonera 2" class="Bool (strict)"("DisabledEnum"=T2."Disabled" ("Disabled")) -> ()  [unwired: 2 in, 2 out]
          }
        }
      }
      event "Botonera 3": Value Change {
        n407 = event-data() -> ()  [unwired: 1 in, 6 out]
        n408 = flat-sequence {
          frame #0 {
            n409 = local read "Subiendo"() -> (w504:bool)
            n410 = case shown="True" w504 {
              tunnel: "Botonera 3" -> [w505 w506]
              frame False {
                n411 = local write "Piso 3_Bajar"(w505) -> ()
              }
              frame True {
                n412 = local write "Piso 3_Subir"(w506) -> ()
              }
            }
          }
          frame #1 {
            n413 = property on="Botonera 3" class="Bool (strict)"("DisabledEnum"=T2."Disabled" ("Disabled")) -> ()  [unwired: 2 in, 2 out]
          }
        }
      }
      event "Botonera 4": Value Change {
        n414 = event-data() -> ()  [unwired: 1 in, 6 out]
        n415 = flat-sequence {
          frame #0 {
            n416 = local write "Piso 4_Bajar"("Botonera 4") -> ()
          }
          frame #1 {
            n417 = property on="Botonera 4" class="Bool (strict)"("DisabledEnum"=T2."Disabled" ("Disabled")) -> ()  [unwired: 2 in, 2 out]
          }
        }
      }
    }
  }
  n418 = local write "Botonera 4"(w3) -> ()
  n419 = local write "Botonera 1"(w3) -> ()
  n420 = local write "Botonera 2"(w3) -> ()
  n421 = local write "Botonera 3"(w3) -> ()
  n422 = Wait (ms)(milliseconds to wait=u32 100) -> ()  [unwired: 1 out]
  "Puerta" <- 8 ("Puerta")
  "Posicion_asensor" <- 100 ("Posicion_asensor")
